vi "make tiff path.vi"(8 "error in (no error)":errorcluster, 10 "current cxd":string, 11 "Trace in":refnum<class "Trace.lvclass">) -> (0 "error out":errorcluster, 3 "Trace out":refnum<class "Trace.lvclass">)   [LabVIEW 2012, in "Trace.lvclass"]
uses:
  Trace.lvclass
  Trace.lvclass/Trace.ctl
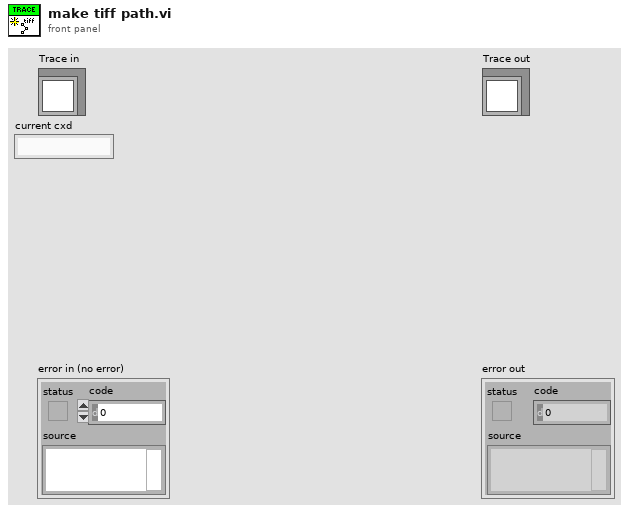
[diagram p1: front panel]
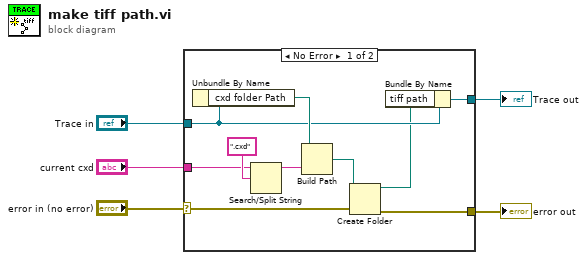
[diagram p0: block diagram]
diagram:
  n1 = case shown="No Error" "error in (no error)" {
    selector: "error in (no error)" -> [w11 w17]
    tunnel: [w6 w17] -> w4
    tunnel: [w8 w16] -> w2
    tunnel: "Trace in" -> [w9 w16]
    tunnel: "current cxd" -> [w14 _]
    frame No Error {
      n2 = Unbundle By Name(w9) -> ("cxd folder Path"=w13:path)
      n3 = Search/Split String(string=w14, search string/char (-)=".cxd") -> (substring before match=w12:string)  [unwired: 1 in, 2 out]
      n4 = Build Path(base path=w13, name or relative path=w12) -> (appended path=w10:path)
      n5 = Create Folder(path (use dialog)=w10, error in=w11) -> (created path=w7:path, error out=w6:errorcluster)  [unwired: 1 in, 1 out]
      n6 = Bundle By Name(cluster=w9, "tiff path"=w7) -> (w8:refnum<class "Trace.lvclass">)
    }
    frame Error {
    }
  }
  "error out" <- w4
  "Trace out" <- w2
